vi "disable_motor.vi"(8 "error in (no error)":errorcluster caption="错误输入（无错误）", 11 "StepMotor输入":refnum<class "StepMotor.lvclass">) -> (0 "error out":errorcluster caption="错误输出", 3 "StepMotor输出":refnum<class "StepMotor.lvclass">)   [LabVIEW 2016, in "MotionControl_UFO_3DOF.lvlib" / "StepMotor.lvclass"]
uses:
  <userlib>/MotionControl_UFO_3DOF/StepMotor/StepMotor.lvclass
  <userlib>/MotionControl_UFO_3DOF/StepMotor/StepMotor.lvclass/StepMotor.ctl
  <userlib>/UISimCanFunc_wrapper/UISimCanFunc_wrapper.lvlib
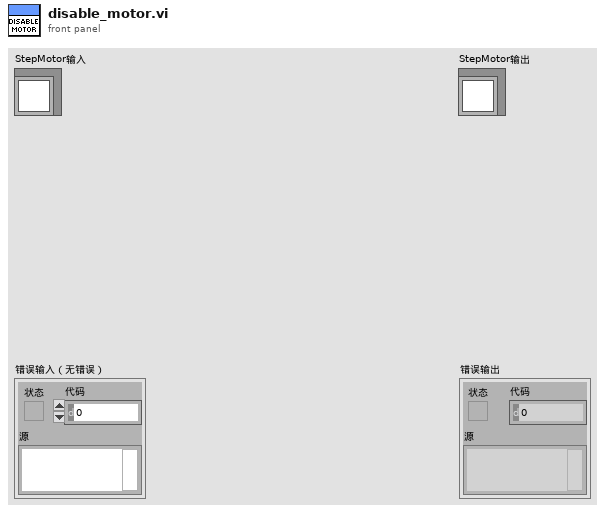
[diagram p1: front panel]
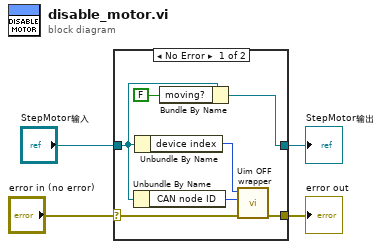
[diagram p0: block diagram]
diagram:
  n1 = case shown="No Error" "error in (no error)" {
    selector: "error in (no error)" -> [w9 w12]
    tunnel: [w8 w12] -> w3
    tunnel: [w6 w13] -> w1
    tunnel: "StepMotor输入" -> [w7 w13]
    frame No Error {
      n2 = Unbundle By Name(w7) -> ("CAN node ID"=w10:u32)
      n3 = Unbundle By Name(w7) -> ("device index"=w11:u32)
      n4 = Bundle By Name(cluster=w7, "moving?"=FALSE) -> (w6:refnum<class "StepMotor.lvclass">)
      n5 = call <userlib>:"Uim OFF wrapper.vi"("error in (no error)"=w9, "dwCanNodeId"=w10, "dwDevIndex"=w11) -> ("error out"=w8:errorcluster)  [unwired: 6 in, 2 out]
    }
    frame Error {
    }
  }
  "error out" <- w3
  "StepMotor输出" <- w1
